vi "OVA_Global_Vars.vi"() -> ()   [LabVIEW 2024]
panel:
  in  "Interferometric DeciFactor":dbl=1.0 format="%.2f"
  in  "GPIB Command?":bool
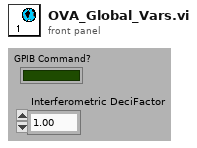
[diagram p1: front panel]
diagram:
